vi "获取两位小时数.vi"() -> (1 "两位数时间":string, 2 "当前时间":string)   [LabVIEW 2017]
panel:
  in  "日期格式":string="/"
  in  "时间标识":timestamp
  out "初始时间":string
  in  "设置初始时间":string
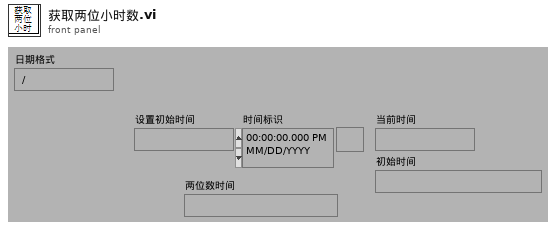
[diagram p1: front panel]
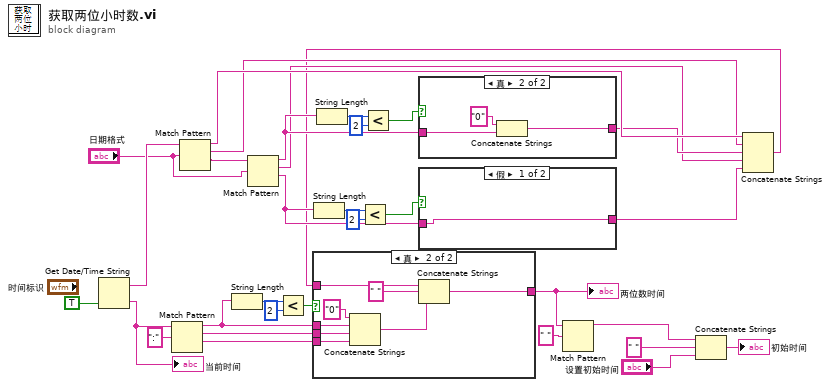
[diagram p0: block diagram]
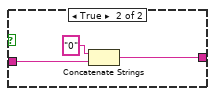
[diagram p2: hidden frame]
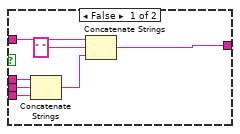
[diagram p4: hidden frame]
diagram:
  n1 = Get Date/Time String(want seconds? (F)=TRUE ("需要秒？(F)")) -> (date string=w17:string, time string=w25:string)  [unwired: 2 in]
  "当前时间" <- w25
  n2 = Match Pattern(string=w25, regular expression=":" ("正则表达式")) -> (before substring=w30:string, match substring=w31:string, after substring=w32:string)  [unwired: 1 in, 1 out]
  n3 = Match Pattern(string=w17, regular expression="日期格式") -> (before substring=w8:string, match substring=w7:string, after substring=w18:string)  [unwired: 1 in, 1 out]
  n4 = String Length(string=w30) -> (length=w27:i32)
  n5 = Match Pattern(string=w18, regular expression="日期格式") -> (before substring=w10:string, match substring=w5:string, after substring=w9:string)  [unwired: 1 in, 1 out]
  n6 = Less?(x=w27, y=2) -> (x < y?=w29:bool)
  n7 = String Length(string=w9) -> (length=w13:i32)
  n8 = String Length(string=w10) -> (length=w16:i32)
  n9 = Less?(x=w13, y=2) -> (x < y?=w11:bool)
  n10 = Less?(x=w16, y=2) -> (x < y?=w12:bool)
  n11 = case shown="真" w12 {
    tunnel: w10 -> [w33 w35]
    tunnel: [w33 w34] -> w6
    frame False {
    }
    frame True {
      n12 = Concatenate Strings("0" ("字符串"), w35) -> (w34:string)
    }
  }
  n13 = case shown="假" w11 {
    tunnel: w9 -> [w37 w39]
    tunnel: [w37 w38] -> w4
    frame False {
    }
    frame True {
      n14 = Concatenate Strings("0" ("字符串"), w39) -> (w38:string)
    }
  }
  n15 = Concatenate Strings(w8, w7, w6, w5, w4) -> (w3:string)
  n16 = case shown="真" w29 {
    tunnel: w30 -> [w45 w52]
    tunnel: w3 -> [w44 w55]
    tunnel: w31 -> [w42 w51]
    tunnel: w32 -> [w41 w50]
    tunnel: [w43 w48] -> w21
    frame False {
      n17 = Concatenate Strings(w45, w42, w41) -> (w46:string)
      n18 = Concatenate Strings(w44, " " ("字符串"), w46) -> (w43:string)
    }
    frame True {
      n19 = Concatenate Strings("0" ("字符串"), w52, w51, w50) -> (w49:string)
      n20 = Concatenate Strings(w55, " " ("字符串"), w49) -> (w48:string)
    }
  }
  "两位数时间" <- w21
  n21 = Match Pattern(string=w21, regular expression=" " ("字符串")) -> (before substring=w1:string)  [unwired: 1 in, 3 out]
  n22 = Concatenate Strings(w1, " " ("字符串"), "设置初始时间") -> (→"初始时间":string)
